vi "PathToMain.vi"(8 "error in":errorcluster) -> (0 "Error Out":errorcluster, 3 "PathToMain":path)   [LabVIEW 2018, in "AcPwrShared.lvlib"]
doc: "This VI attempts to find the file path location to Main.vi located in the AcPwr Plugin Library. If it cannot find the location it promts the user to manually search and select Main.vi."
uses:
  AcPwrShared.lvlib
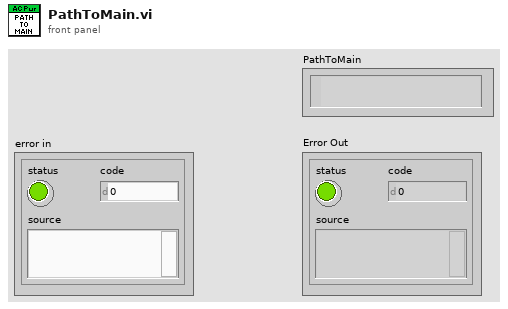
[diagram p1: front panel]
types:
  T1 = enum16{"open", "replace", "create", "open or create", "replace or create", "replace or create with confirmation"}
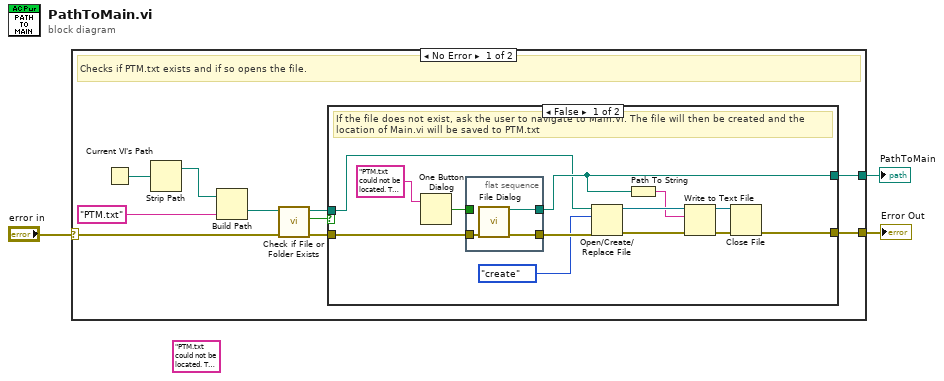
[diagram p0: block diagram]
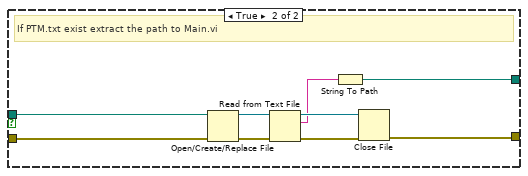
[diagram p2: hidden frame]
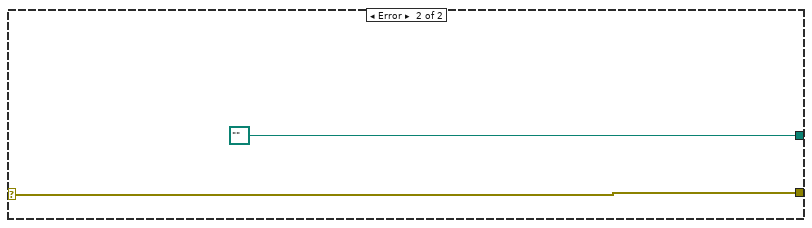
[diagram p3: hidden frame]
diagram:
  (unwired) "PTM.txt could not be located. This file does not exist or is in the wrong location. PTM.txt stores the location of Main.VI. After you've exited this dialog a window file explorer window will appear. Use it to navigate to Main (typically located in C:\\Users\\ico\\Documents\\Projects\\NistPluggableModules\\AcPwr\\AcPwrPlugins\\Common). A new version of PTM.txt will be created and the file path to main will be stored in PTM.txt " ("name or relative path")
  n1 = case shown="No Error" "error in" {
    selector: "error in" -> [w11 w40]
    tunnel: [w13 w40] -> w1
    tunnel: [w12 path "" ("selected path")] -> w3
    frame No Error {
      # "Checks if PTM.txt exists and if so opens the file."
      n2 = Current VI's Path() -> (path=w5:path)
      n3 = Strip Path(path=w5) -> (stripped path=w4:path)  [unwired: 1 out]
      n4 = Build Path(base path=w4, name or relative path="PTM.txt") -> (appended path=w6:path)
      n5 = call <vilib>:"Check if File or Folder Exists.vi"("error in (no error)"=w11, "path"=w6) -> ("error out"=w10:errorcluster, "file or folder exists?"=w9:bool, "dup path"=w8:path)  [unwired: 7 in]
      n6 = case shown="False" w9 {
        tunnel: [w18 w32] -> w12
        tunnel: [w21 w34] -> w13
        tunnel: w10 -> [w26 w38]
        tunnel: w8 -> [w17 w31]
        frame False {
          # "If the file does not exist, ask the user to navigate to Main.VI. The file will then be created and the location of Main.vi will be saved to PTM.txt"
          n7 = One Button Dialog(message="PTM.txt could not be located. This file does not exist or is in the wrong location. PTM.txt stores the location of Main.VI. After you've exited this dialog a window file explorer window will appear. Use it to navigate to Main (typically located in C:\\Users\\ico\\Documents\\Projects\\NistPluggableModules\\AcPwr\\AcPwrPlugins\\Common). A new version of PTM.txt will be created and the file path to main will be stored in PTM.txt " ("name or relative path")) -> (true=w15:bool)  [unwired: 1 in]
          n8 = flat-sequence {
            tunnel: w26 -> [w29]
            tunnel: [w28] -> w20
            tunnel: [w27] -> w18
            tunnel: w15 -> [_]
            frame #0 {
              n9 = call "File Dialog"("error in"=w29) -> ("selected path"=w27:path, "error out"=w28:errorcluster)  [unwired: 11 in, 2 out]
            }
          }
          n10 = Open/Create/Replace File(file path (use dialog)=w17, error in=w20, operation (0:open)=T1."create") -> (refnum out=w24:refnum<file>, error out=w25:errorcluster)  [unwired: 3 in, 1 out]
          n11 = Path To String(path=w18) -> (string=w19:string)
          n12 = Write to Text File(file (use dialog)=w24, text=w19, error in=w25) -> (refnum out=w22:refnum<file>, error out=w23:errorcluster)  [unwired: 1 in, 1 out]
          n13 = Close File(refnum=w22, error in=w23) -> (error out=w21:errorcluster)  [unwired: 1 out]
        }
        frame True {
          # "If PTM.txt exist extract the path to Main.vi"
          n14 = Open/Create/Replace File(file path (use dialog)=w31, error in=w38) -> (refnum out=w30:refnum<file>, error out=w37:errorcluster)  [unwired: 4 in, 1 out]
          n15 = Read from Text File(file (use dialog)=w30, error in=w37) -> (refnum out=w35:refnum<file>, text=w33:string, error out=w36:errorcluster)  [unwired: 2 in, 1 out]
          n16 = String To Path(string=w33) -> (path=w32:path)
          n17 = Close File(refnum=w35, error in=w36) -> (error out=w34:errorcluster)  [unwired: 1 out]
        }
      }
    }
    frame Error {
    }
  }
  "PathToMain" <- w3
  "Error Out" <- w1
